vi "Generate LabVIEW FPGA Code for Moving Average Filter.vi"() -> ()   [LabVIEW 2023]
doc: "Demonstrates how to use the DFD FXP MRate Code Generator VI to generate LabVIEW field-programmable gate array (FPGA) code from a fixed-point, moving average (MA) filter.\n\nComplete the following steps to use this VI.\n1) Specify the <B>Filter Settings</B> and <B>Modeling Settings</B>.\n2) Specify a <B>Destination Folder</B> for code generation.\n3) Specify a <B>Filter Name</B> for code generation.\n4) Specify <B># Channels</B> that you want the filter to process.\n5) Specify <B>Open Project?</B> to decide whether to open the generated LabVIEW project or not after code generation.\n6) Run the VI.\n7) Observe the Maximum Input Fs@40 MHz FPGA Clock to obtain information about the processing power of the generated fixed-point MA filter block."
uses:
  <vilib>/addons/Digital Filter Design/_Objects.llb/DFD Multirate Filtering Mode.ctl
  <vilib>/addons/Digital Filter Design/_Objects.llb/DFD FXP MRate Internal Precision Mode.ctl
  <vilib>/addons/Digital Filter Design/NI_DigFilterLicensed.lvlib
panel:
  in  "1/N Gain Settings":T1={"gain processing"=1, "gain word length"=16} {"gain processing" items=["On Target", "On Host"]}
  in  "Filtering Mode":T2=2 items=["No Rate Change", "Interpolation", "Decimation"]
  out "Maximum Input Fs@40 MHz FPGA Clock":dbl format="%#_5p Hz"
  out "lvproj Path":path
  in  "Open Project?":bool=TRUE
  in  "Filter Name":string
  in  "# Channels":i32=1
  in  "Destination Folder":path
  out "Error Message":string
  in  "Output Word Length":i16=16
  in  "Input Word Length":i16=16
  in  "N":i32=16
  # "Select Help>>Show Context Help and move the cursor over the VI icon for more information."
  # "Filter Settings"
  # "Modeling Settings"
  # "Code Generation Settings"
  # "Code Generation Feedback"
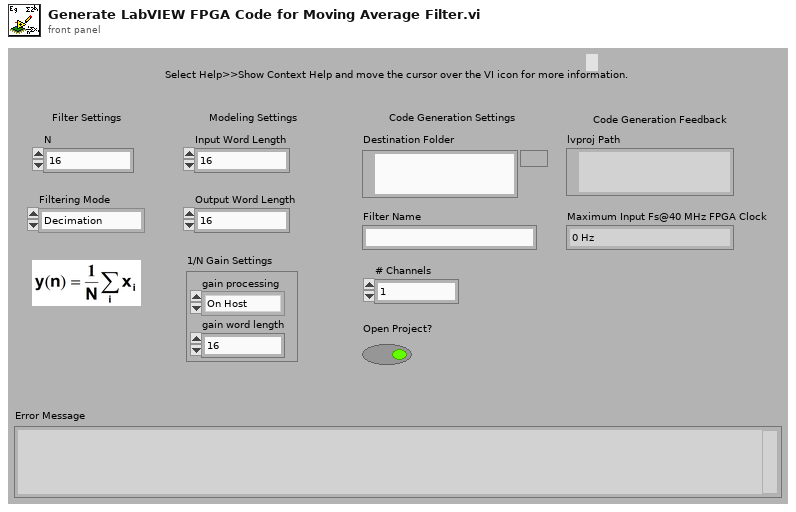
[diagram p1: front panel]
types:
  T1 = cluster{"gain processing":u16, "gain word length":i16}
  T2 = typedef "NI_DigFilterLicensed.lvlib/DFD Multirate Filtering Mode.ctl" = u16
  T3 = typedef "NI_DigFilterLicensed.lvlib/DFD FXP MRate Internal Precision Mode.ctl" = enum16{"Truncated", "Full"}
  T4 = typedef "NI_DigFilterLicensed.lvlib/DFD Multirate Filter Obj.ctl" = cluster{"mMRate_Structure":enum16{"CIC", "FIR", "IIR", "Lattice"}, "mMRate_Mode":T5, "mMRate_Factor":i32, "mMRate_FIRParams":cluster{"mMRate_FIR_H":dbl[], "mMRate_FIR_IsNyquist?":bool, "mMRate_FIR_IsSymmetric?":bool}, "mMRate_CICParams":cluster{"mMRate_CIC_#Stage":i32, "mMRate_CIC_Lag":i32, "mMRate_CIC_Type":enum16{"Lowpass", "Highpass"}}, "mMRate_Order":i32, "mMRate_Version":string, "mMRate_Comments":string, "mMRate_RationalFactor":cluster{"mMRate_L":i32, "mMRate_M":i32}, "mMRate_Fs":dbl, "mMRate_Quantized?":bool, "mMRate_QFilterGain":dbl, "mMRate_CoefWl":i16, "mMRate_Scaling":cluster{"mMRate_ScaleByPowerOf2?":bool, "mMRate_ScaleType":T6}, "mMRate_InputWl":i16, "mMRate_OutputWl":i16, "mMRate_OutputMode":T7, "mMRate_MultMode":T8, "mMRate_BitPruning":bool, "mMRate_GainWl":i16, "mMRate_OutputFwl":i16, "mMRate_SumIwl":i16, "mMRate_InputIwl ":i16, "mMRate_SumWl":i16, "mMRate_CoefIwl":i16}
  T5 = typedef "NI_DigFilterLicensed.lvlib/DFD Multirate Mode.ctl" = i16
  T6 = typedef "NI_DigFilterLicensed.lvlib/DFD Coef Norm Type.ctl" = enum16{"No Norm", "Time Domain 1-Norm", "Time Domain 2-Norm", "Time Domain Inf-Norm"}
  T7 = typedef "NI_DigFilterLicensed.lvlib/DFD Round-off Mode.ctl" = enum16{"Nearest", "Truncation"}
  T8 = typedef "NI_DigFilterLicensed.lvlib/DFD FXP MRate Multiply Mode.ctl" = enum16{"Truncated", "Full"}
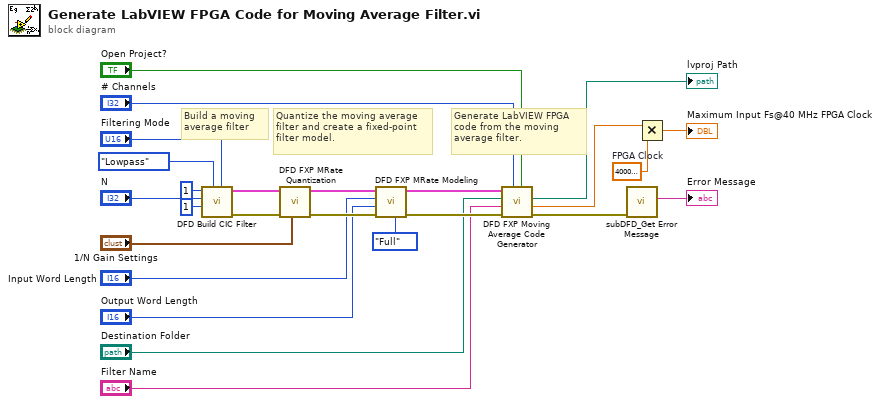
[diagram p0: block diagram]
diagram:
  w1 = 40000000.0  # FPGA Clock
  # "Generate LabVIEW FPGA \ncode from the moving \naverage filter."
  # "Quantize the moving average\nfilter and create a fixed-point\nfilter model."
  # "Build a moving \naverage filter"
  n1 = call <vilib>:"DFD Build CIC Filter.vi"("filtering mode"="Filtering Mode", "filter type"=enum16{"Lowpass", "Highpass"}."Lowpass", "differential delay"=1 ("lag"), "factor"="N", "# stages"=1) -> ("error out"=w19:errorcluster, "CIC filter out"=w20:T4)  [unwired: 2 in, 3 out]
  n2 = call <vilib>:"DFD FXP MRate Quantization.vi"("gain settings"="1/N Gain Settings", "error in (no error)"=w19, "multirate filter in"=w20) -> ("error out"=w16:errorcluster, "multirate filter out"=w17:T4)  [unwired: 3 in, 4 out]
  n3 = call <vilib>:"DFD FXP MRate Modeling.vi"("internal precision"=DFD_FXP_MRate_Internal_Precision_Mode."Full", "error in (no error)"=w16, "output word length"="Output Word Length", "input word length"="Input Word Length", "multirate filter in"=w17) -> ("error out"=w12:errorcluster, "multirate filter out"=w13:T4)  [unwired: 3 in, 2 out]
  n4 = call <vilib>:"DFD FXP Moving Average Code Generator.vi"("open project? (F)"="Open Project?", "# channels"="# Channels", "error in (no error)"=w12, "filter name"="Filter Name", "destination folder"="Destination Folder", "moving average filter"=w13) -> ("error out"=w4:errorcluster, "sampling frequency/FPGA clock"=w6:dbl, "lvproj path"=→"lvproj Path":path)  [unwired: 1 in, 2 out]
  n5 = call <vilib>:"subDFD_Get Error Message.vi"("error in (no error)"=w4) -> ("Error Message"=→"Error Message":string)  [unwired: 10 out]
  n6 = Multiply(x=w6, y=w1) -> (x*y=→"Maximum Input Fs@40 MHz FPGA Clock":dbl)
